vi "Ultrasonic sensor.vi"() -> ()   [LabVIEW 2022 SP3]
uses:
  <vilib>/DAQmx/write.llb/DAQmx Write (Digital Bool 1Line 1Point).vi
  <vilib>/DAQmx/read.llb/DAQmx Read (Analog Wfm 1Chan NSamp).vi
  <vilib>/DAQmx/create/channels.llb/DAQmx Create Channel (AI-Voltage-Basic).vi
  <vilib>/DAQmx/configure/timing.llb/DAQmx Timing (Sample Clock).vi
  <vilib>/DAQmx/create/channels.llb/DAQmx Create Channel (DO-Digital Output).vi
  <vilib>/DAQmx/miscellaneous.llb/DAQmx Fill In Error Info.vi
panel:
  out "water level detector":bool
  in  "ultrasonic digital output channel":tag
  in  "stop 3":bool
  in  "ultrasonic analog input channel":tag
  out "Waveform Graph":waveform(dbl)(graph)
  out "No of samples":dbl
  out "Distance":dbl
  # "ULTRASONIC SENSOR"
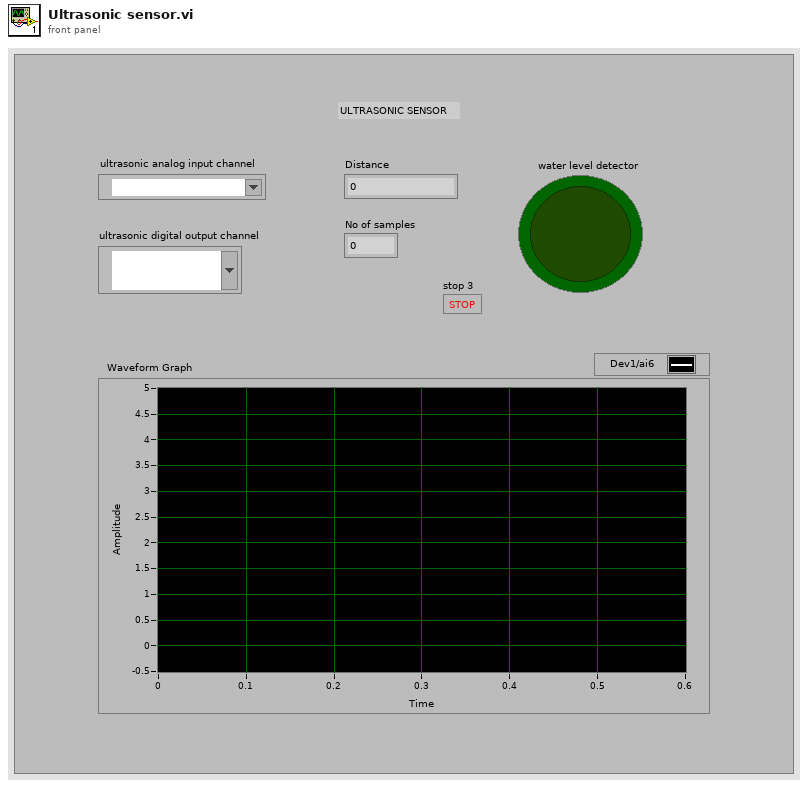
[diagram p1: front panel]
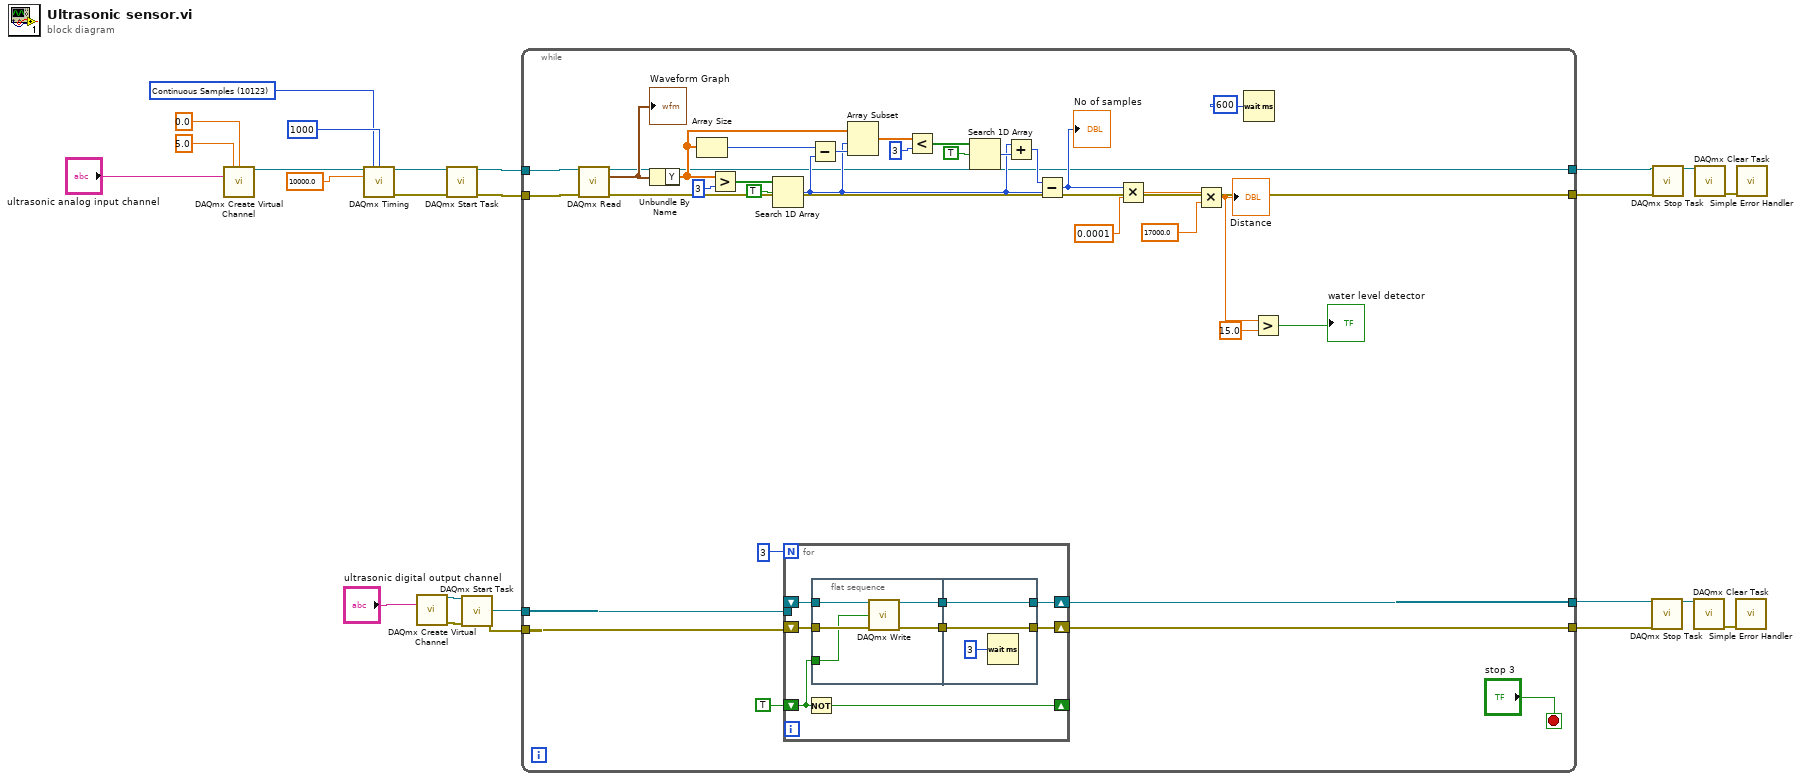
[diagram p0: block diagram]
diagram:
  w17 = 10123 items=["Finite Samples"=10178, "Continuous Samples"=10123, "Hardware Timed Single Point"=12522] ("sample mode")
  n1 = call-poly <vilib>:"DAQmx Create Virtual Channel.vi"("maximum value"=5.0, "minimum value"=0.0, "physical channels"="ultrasonic analog input channel") -> ("task out"=w22:refnum<k21>)  [unwired: 11 in, 1 out]
  n2 = call-poly <vilib>:"DAQmx Timing.vi"("task/channels in"=w22, "sample mode"=w17, "samples per channel"=1000, "rate"=10000.0) -> ("task out"=w23:refnum<k21>, "error out"=w15:errorcluster)  [unwired: 10 in]
  n3 = call-poly <vilib>:"DAQmx Create Virtual Channel.vi"("lines"="ultrasonic digital output channel") -> ("task out"=w8:refnum<k21>, "error out"=w7:errorcluster)  [unwired: 13 in]
  n4 = call <vilib>:"DAQmx Start Task.vi"("task/channels in"=w23, "error in"=w15) -> ("task out"=w16:refnum<k21>, "error out"=w14:errorcluster)  [unwired: 12 in]
  n5 = call <vilib>:"DAQmx Start Task.vi"("task/channels in"=w8, "error in"=w7) -> ("task out"=w6:refnum<k21>, "error out"=w5:errorcluster)  [unwired: 12 in]
  n6 = while {
    tunnel: w16 -> [w57]
    tunnel: w6 -> [w36]
    tunnel: w14 -> [w56]
    tunnel: w5 -> [w35]
    tunnel: [w34] -> w11
    tunnel: [w33] -> w10
    tunnel: [w30] -> w2
    tunnel: [w29] -> w1
    stop <- "stop 3" stop-if-true
    n7 = call-poly <vilib>:"DAQmx Read.vi"("task/channels in"=w57, "error in"=w56) -> ("task out"=w30:refnum<k21>, "data"=w31:waveform(dbl), "error out"=w29:errorcluster)  [unwired: 11 in]
    "Waveform Graph" <- w31
    n8 = Unbundle By Name(w31) -> ("Y"=w51:dbl[])
    n9 = Array Size(array=w51) -> (size(s)=w50:i32)
    n10 = Greater?(x=w51, y=3) -> (0:w54:bool[])
    n11 = Search 1D Array(1D array=w54, element=TRUE) -> (index of element=w44:i32)  [unwired: 1 in]
    n12 = for {
      N: 3 -> [_]
      shift-right: [w60] -> w34
      shift-left: _ -> [w63]
      shift-right: [w61] -> w33
      shift-left: w35 -> [w62]
      shift-right: [w59] -> _
      shift-left: TRUE -> [w58]
      tunnel: w36 -> [_]
      n13 = Not(x=w58) -> (.not. x?=w59:bool)
      n14 = flat-sequence {
        tunnel: w63 -> [w70]
        tunnel: w62 -> [w69]
        tunnel: [w68] -> w65
        tunnel: [w67] -> w64
        tunnel: w58 -> [w66]
        tunnel: w65 -> [w71]
        tunnel: w64 -> [w72]
        tunnel: [w72] -> w61
        tunnel: [w71] -> w60
        frame #0 {
          n15 = call-poly <vilib>:"DAQmx Write.vi"("task/channels in"=w70, "data"=w66, "error in"=w69) -> ("task out"=w68:refnum<k21>, "error out"=w67:errorcluster)  [unwired: 10 in, 1 out]
        }
        frame #1 {
          n16 = Wait (ms)(milliseconds to wait=u32 3) -> ()  [unwired: 1 out]
        }
      }
    }
    n17 = Subtract(x=w50, y=w44) -> (x-y=w49:i32)
    n18 = Array Subset(array=w51, index=w44, length=w49) -> (w48:dbl[])
    n19 = Less?(x=w48, y=3) -> (x < y?=w46:bool[])
    n20 = Search 1D Array(1D array=w46, element=TRUE) -> (index of element=w45:i32)  [unwired: 1 in]
    n21 = Add(x=w44, y=w45) -> (x+y=w43:i32)
    n22 = Subtract(x=w43, y=w44) -> (x-y=w41:i32)
    "No of samples" <- w41
    n23 = Multiply(x=w41, y=0.0001) -> (x*y=w40:dbl)
    n24 = Multiply(x=w40, y=17000.0) -> (x*y=w26:dbl)
    "Distance" <- w26
    n25 = Wait (ms)(milliseconds to wait=u32 600) -> ()  [unwired: 1 out]
    n26 = Greater?(x=w26, y=15.0) -> (0:→"water level detector":bool)
  }
  n27 = call <vilib>:"DAQmx Stop Task.vi"("task/channels in"=w11, "error in"=w10) -> ("task out"=w13:refnum<k21>)  [unwired: 12 in, 1 out]
  n28 = call <vilib>:"DAQmx Stop Task.vi"("task/channels in"=w2, "error in"=w1) -> ("task out"=w4:refnum<k21>)  [unwired: 12 in, 1 out]
  n29 = call <vilib>:"DAQmx Clear Task.vi"("task in"=w13) -> ("error out"=w12:errorcluster)  [unwired: 14 in]
  n30 = call <vilib>:"DAQmx Clear Task.vi"("task in"=w4) -> ("error out"=w3:errorcluster)  [unwired: 14 in]
  n31 = call <vilib>:"Simple Error Handler.vi"("error in (no error)"=w12) -> ()  [unwired: 4 in, 5 out]
  n32 = call <vilib>:"Simple Error Handler.vi"("error in (no error)"=w3) -> ()  [unwired: 4 in, 5 out]
